vi "Pre Launch Init.vi"(11 "Nested in":refnum<class "Contabilidad.lvclass">) -> (0 "error out":errorcluster, 3 "Nested out":refnum<class "Contabilidad.lvclass">)   [LabVIEW 2020, in "Contabilidad.lvlib" / "Contabilidad.lvclass"]
doc: "(<B>Filename</B>: Actor Framework.lvlib:Actor.lvclass:Pre Launch Init.vi)\n\nDefines behavior that occurs after the Launch Nested Actor method is invoked but before the actor's Actor Core method begins running.\n\nBy default, this method does nothing. A descendant class may override it to define behavior."
uses:
  Contabilidad.lvclass
  C:/Program Files (x86)/National Instruments/LabVIEW 2020/vi.lib/ActorFramework/Actor/Actor.lvclass
  Contabilidad.lvclass/Contabilidad.ctl
  <vilib>/ActorFramework/Actor/Actor.lvclass/Actor.ctl
  <vilib>/ActorFramework/Message Enqueuer/Message Enqueuer.lvclass/Message Enqueuer.ctl
  <vilib>/ActorFramework/Message Enqueuer/Enqueue.vi
  <vilib>/ActorFramework/Message Enqueuer/Init from Existing Queue.vi
  Contabilidad Messages/Create Table Database Msg/Create Table Database Msg.lvclass
  C:/Program Files (x86)/National Instruments/LabVIEW 2020/vi.lib/ActorFramework/Message/Message.lvclass
  <vilib>/ActorFramework/Message Priority Queue/Priority Enqueue.vi
  <vilib>/ActorFramework/Message Enqueuer/Message Enqueuer.lvclass
  <vilib>/ActorFramework/Actor/Actor.lvclass
  C:/Users/HP/Desktop/Salma_Aguayo/Contabilidad/Contabilidad.lvclass
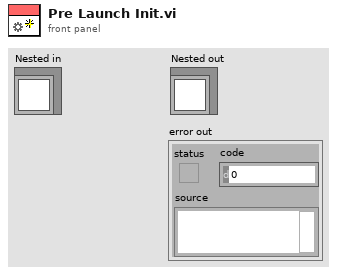
[diagram p1: front panel]
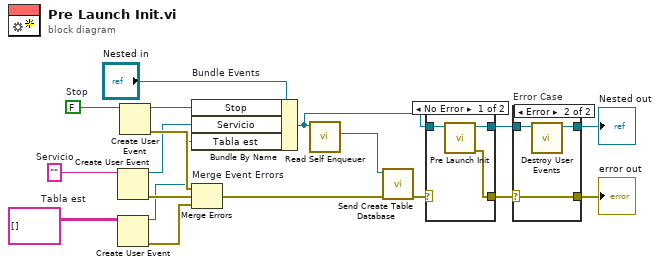
[diagram p0: block diagram]
diagram:
  w3 = string[][] []  # Tabla est
  w10 = ""  # Servicio
  w17 = FALSE  # Stop
  n1 = Create User Event(user event datatype=w10) -> (user event=w9:refnum<user-event>, error out=w8:errorcluster)  [unwired: 1 in]
  n2 = Create User Event(user event datatype=w3) -> (user event=w1:refnum<user-event>, error out=w2:errorcluster)  [unwired: 1 in]
  n3 = Create User Event(user event datatype=w17) -> (user event=w14:refnum<user-event>, error out=w16:errorcluster)  [unwired: 1 in]
  n4 = Bundle By Name "Bundle Events"(cluster="Nested in", "Stop"=w14, "Servicio"=w9, "Tabla est"=w1) -> (w4:refnum<class "Contabilidad.lvclass">)
  n5 = Merge Errors "Merge Event Errors"(w16, w8, w2) -> (w6:errorcluster)
  n6 = call <vilib>:"Read Self Enqueuer.vi"("Actor"=w4) -> ("Self Enqueuer"=w5:refnum<class "Message Enqueuer.lvclass">)  [unwired: 10 in]
  n7 = call "Send Create Table Database.vi"("error in (no error)"=w6, "Message Enqueuer"=w5) -> ("error out"=w7:errorcluster)  [unwired: 8 in, 1 out]
  n8 = case shown="No Error" w7 {
    selector: w7 -> [_ w23]
    tunnel: [w21 w22] -> w12
    tunnel: w4 -> [w20 w22]
    tunnel: [w19 w23] -> w11
    frame No Error {
      n9 = call-parent "Pre Launch Init.vi"("Actor in"=w20) -> ("error out"=w19:errorcluster, "Actor out"=w21:refnum<class "Contabilidad.lvclass">)  [unwired: 9 in]
    }
    frame Error {
    }
  }
  n10 = case "Error Case" shown="Error" w11 {
    selector: w11 -> [w24 w28]
    tunnel: w12 -> [w25 w27]
    tunnel: [w25 w26] -> w15
    tunnel: [w24 w28] -> w13
    frame No Error {
    }
    frame Error {
      n11 = call "Destroy User Events.vi"("UI Template in"=w27) -> ("UI Template out"=w26:refnum<class "Contabilidad.lvclass">)  [unwired: 10 in]
    }
  }
  "error out" <- w13
  "Nested out" <- w15
